vi "Kernel32 GetLastError.vi"(8 "error in (no error)":errorcluster, 11 "Message":string) -> (0 "error out":errorcluster)   [LabVIEW 2011]
uses:
  kernel32.dll
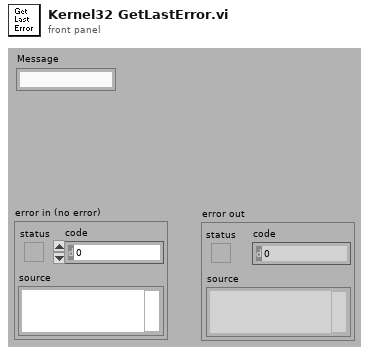
[diagram p1: front panel]
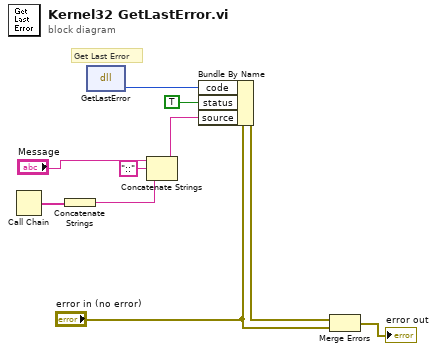
[diagram p0: block diagram]
diagram:
  # "Get Last Error"
  n1 = Call Chain() -> (call chain=w6:string[])
  n2 = Concatenate Strings(w6) -> (w4:string)
  n3 = dll-call lib="kernel32.dll" fn="GetLastError"() -> ("return type"=w10:u16)  [unwired: 3 in, 2 out]
  n4 = Concatenate Strings("Message", "::" ("string"), w4) -> (w2:string)
  n5 = Bundle By Name(cluster="error in (no error)", "code"=w10, "status"=TRUE, "source"=w2) -> (w8:errorcluster)
  n6 = Merge Errors(w8, "error in (no error)") -> (→"error out":errorcluster)
